vi "FlatToRichexternal_driver_wrapper_ReadResponse.vi"(5 "OutputClusterType":T1, 11 "InputCluster":T2) -> (3 "OutputCluster":T1)   [LabVIEW 2020, in "Instrument Interaction Client.lvlib"]
uses:
  Instrument Interaction Client.lvlib
  external_driver_wrapper_ReadResponse_Flat.ctl
  external_driver_wrapper_ReadResponse.ctl
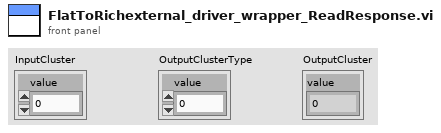
[diagram p1: front panel]
types:
  T1 = typedef "Instrument Interaction Client.lvlib/external_driver_wrapper_ReadResponse.ctl" = cluster{"value":dbl}
  T2 = typedef "Instrument Interaction Client.lvlib/external_driver_wrapper_ReadResponse_Flat.ctl" = cluster{"value":dbl}
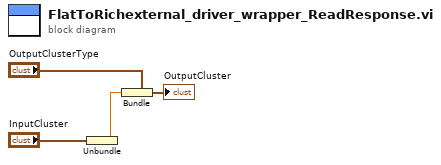
[diagram p0: block diagram]
diagram:
  n1 = Unbundle "Unbundle"("InputCluster") -> ("value"=w1:dbl)
  n2 = Bundle "Bundle"(cluster="OutputClusterType", "value"=w1) -> (→"OutputCluster":T1)
